vi "Update_trial_state.vi"(6 "Next state":string, 11 "Sequence state in":T1={"Current state"="Waiting for trigger", "Response states"={"Response"=FALSE, "Response past threshold"=FALSE, "Response in window"=FALSE, "Punished response"=FALSE, "Response window"=FALSE}, "Next sequence"={"Name"="", "Trigger"=0, "Stimulus interval"=0.0, "Stimuli"=[], "Reward condition"=0}, "Stimuli left"=[]}) -> (3 "Sequence state out":T1={"Current state"="Waiting for trigger", "Response states"={"Response"=FALSE, "Response past threshold"=FALSE, "Response in window"=FALSE, "Punished response"=FALSE, "Response window"=FALSE}, "Next sequence"={"Name"="", "Trigger"=0, "Stimulus interval"=0.0, "Stimuli"=[], "Reward condition"=0}, "Stimuli left"=[]})   [LabVIEW 2016]
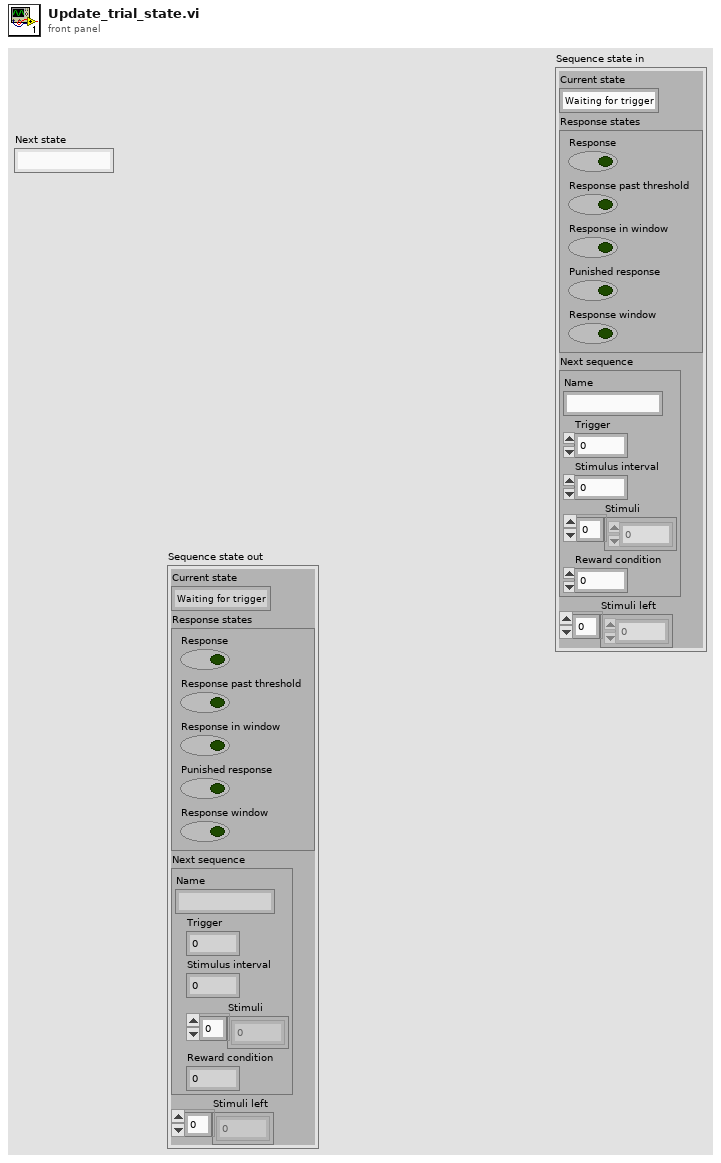
[diagram p1: front panel]
types:
  T1 = cluster{"Current state":string, "Response states":cluster{"Response":bool, "Response past threshold":bool, "Response in window":bool, "Punished response":bool, "Response window":bool}, "Next sequence":cluster{"Name":string, "Trigger":u16, "Stimulus interval":dbl, "Stimuli":i32[], "Reward condition":u16}, "Stimuli left":i32[]}
  T2 = cluster{"Name":string, "Trigger":u16, "Stimulus interval":dbl, "Stimuli":i32[], "Reward condition":u16}
  T3 = cluster{"Response":bool, "Response past threshold":bool, "Response in window":bool, "Punished response":bool, "Response window":bool}
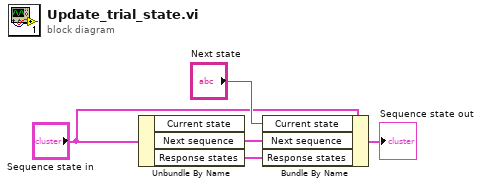
[diagram p0: block diagram]
diagram:
  n1 = Unbundle By Name("Sequence state in") -> ("Next sequence"=w3:T2, "Response states"=w4:T3)  [unwired: 1 out]
  n2 = Bundle By Name(cluster="Sequence state in", "Current state"="Next state", "Next sequence"=w3, "Response states"=w4) -> (→"Sequence state out":T1)
